vi "Open Actor Core Input Terminal Ref.vi"(10 "TopLevelDiagram in":refnum<vi>) -> (0 "error out":errorcluster, 1 "VI Input Found?":bool, 3 "Actor Input ControlTerminal":refnum<vi>)   [LabVIEW 2020, in "Add to Private Data.lvlib"]
uses:
  Add to Private Data.lvlib
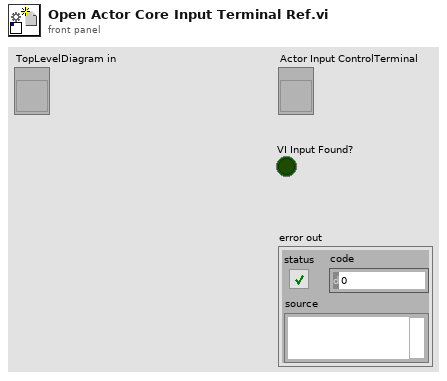
[diagram p1: front panel]
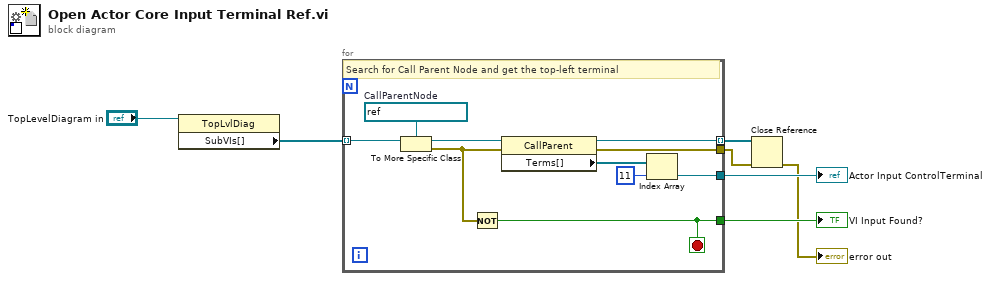
[diagram p0: block diagram]
diagram:
  n1 = property on="Property Node" class="TopLvlDiag"(reference="TopLevelDiagram in") -> ("SubVIs[]"=w7:refnum<vi>[])  [unwired: 1 in, 2 out]
  n2 = for {
    tunnel: w7 -> [w17] mode=indexing
    tunnel: [w10] -> w5
    tunnel: [w12] -> w4
    tunnel: [w9] -> w3 mode=indexing
    tunnel: [w8] -> w2
    stop <- w10 stop-if-true
    w16 = refnum<vi> refnum  # CallParentNode
    # "Search for Call Parent Node and get the top-left terminal"
    n3 = To More Specific Class(target class=w16, reference=w17) -> (specific class reference=w15:refnum<vi>, error out=w11:errorcluster)  [unwired: 1 in]
    n4 = Not(x=w11) -> (.not. x?=w10:bool)
    n5 = property on="Property Node" class="CallParent"(reference=w15, error in=w11) -> (reference out=w9:refnum<vi>, error out=w8:errorcluster, "Terms[]"=w14:refnum<vi>[])
    n6 = Index Array(array=w14, index=11) -> (element=w12:refnum<vi>)
  }
  "Actor Input ControlTerminal" <- w4
  "VI Input Found?" <- w5
  n7 = Close Reference(reference=w3, error in (no error)=w2) -> (error out=→"error out":errorcluster)
